vi "WAIT.vi"(10 "argv":string[](array[string]), 11 "args":u8) -> ()   [LabVIEW 2012]
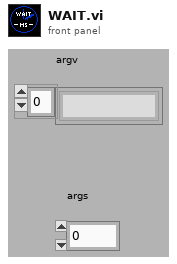
[diagram p1: front panel]
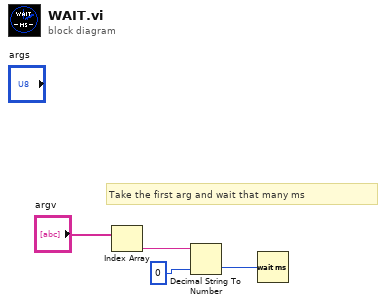
[diagram p0: block diagram]
diagram:
  # "Take the first arg and wait that many ms"
  n1 = Index Array(array="argv") -> (element=w3:string)  [unwired: 1 in]
  n2 = Decimal String To Number(string=w3, default (0L)=u32 0 ("milliseconds to wait")) -> (number=w1:u32)  [unwired: 2 out]
  n3 = Wait (ms)(milliseconds to wait=w1) -> ()  [unwired: 1 out]
